vi "Fixed-Point Multirate Filter Modeling and Simulation.vi"() -> ()   [LabVIEW 2023]
doc: "Demonstrates how to use the DFD FXP MRate Modeling VI and the DFD FXP MRate Simulation VI to model and simulate the behavior of a fixed-point multirate filter, respectively."
uses:
  <vilib>/addons/Digital Filter Design/_Objects.llb/DFD Quantization Settings.ctl
  <vilib>/addons/Digital Filter Design/_Objects.llb/DFD Quantization Sources.ctl
  <vilib>/addons/Digital Filter Design/Design.llb/DFD MRate Filter Design (Integer).vi
  <vilib>/addons/Digital Filter Design/FXPMRateSim.llb/DFD FXP MRate Simulation (DBL).vi
  <vilib>/addons/Digital Filter Design/Multirate.llb/DFD MRate Filtering (Array).vi
  <vilib>/Analysis/NI_AALBase.lvlib
  <vilib>/addons/Digital Filter Design/NI_DigFilterLicensed.lvlib
  <vilib>/Analysis/NI_AALPro.lvlib
panel:
  out "MSE":dbl format="%.6g"
  out "Error Message":string
  out "Filtered Signals":dbl[][](graph)
  in  "Output Word Length":i16=16
  in  "Input Word Length":i16=16
  in  "Coefficients Word Length":i16=16
  in  "Source":enum16{"Sine", "Random Noise"}(ring)
  in  "Number of Samples":i32=128
  # "Select Help>>Show Context Help and move the cursor over the VI icon for more information."
  # "Quantization Setting"
  # "Signal Settings"
  # "Modeling Settings"
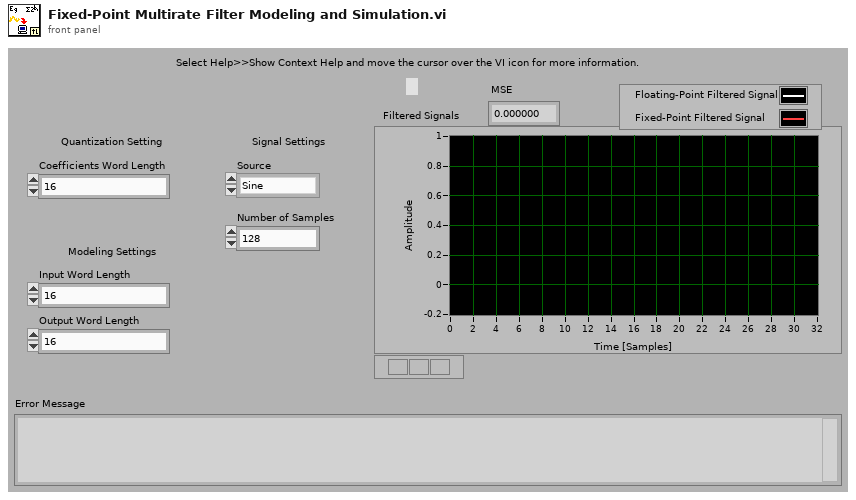
[diagram p1: front panel]
types:
  T1 = typedef "NI_DigFilterLicensed.lvlib/DFD Quantization Settings.ctl" = cluster{"source":T2, "wl":i16, "iwl":i16, "overflow mode":enum16{"Saturation", "Wrap"}, "rounding mode":enum16{"Nearest", "Truncation"}, "signed?":bool}
  T2 = typedef "NI_DigFilterLicensed.lvlib/DFD Quantization Sources.ctl" = u16
  T3 = typedef "NI_DigFilterLicensed.lvlib/DFD Multirate Filter Obj.ctl" = cluster{"mMRate_Structure":enum16{"CIC", "FIR", "IIR", "Lattice"}, "mMRate_Mode":T4, "mMRate_Factor":i32, "mMRate_FIRParams":cluster{"mMRate_FIR_H":dbl[], "mMRate_FIR_IsNyquist?":bool, "mMRate_FIR_IsSymmetric?":bool}, "mMRate_CICParams":cluster{"mMRate_CIC_#Stage":i32, "mMRate_CIC_Lag":i32, "mMRate_CIC_Type":enum16{"Lowpass", "Highpass"}}, "mMRate_Order":i32, "mMRate_Version":string, "mMRate_Comments":string, "mMRate_RationalFactor":cluster{"mMRate_L":i32, "mMRate_M":i32}, "mMRate_Fs":dbl, "mMRate_Quantized?":bool, "mMRate_QFilterGain":dbl, "mMRate_CoefWl":i16, "mMRate_Scaling":cluster{"mMRate_ScaleByPowerOf2?":bool, "mMRate_ScaleType":T5}, "mMRate_InputWl":i16, "mMRate_OutputWl":i16, "mMRate_OutputMode":T6, "mMRate_MultMode":T7, "mMRate_BitPruning":bool, "mMRate_GainWl":i16, "mMRate_OutputFwl":i16, "mMRate_SumIwl":i16, "mMRate_InputIwl ":i16, "mMRate_SumWl":i16, "mMRate_CoefIwl":i16}
  T4 = typedef "NI_DigFilterLicensed.lvlib/DFD Multirate Mode.ctl" = i16
  T5 = typedef "NI_DigFilterLicensed.lvlib/DFD Coef Norm Type.ctl" = enum16{"No Norm", "Time Domain 1-Norm", "Time Domain 2-Norm", "Time Domain Inf-Norm"}
  T6 = typedef "NI_DigFilterLicensed.lvlib/DFD Round-off Mode.ctl" = enum16{"Nearest", "Truncation"}
  T7 = typedef "NI_DigFilterLicensed.lvlib/DFD FXP MRate Multiply Mode.ctl" = enum16{"Truncated", "Full"}
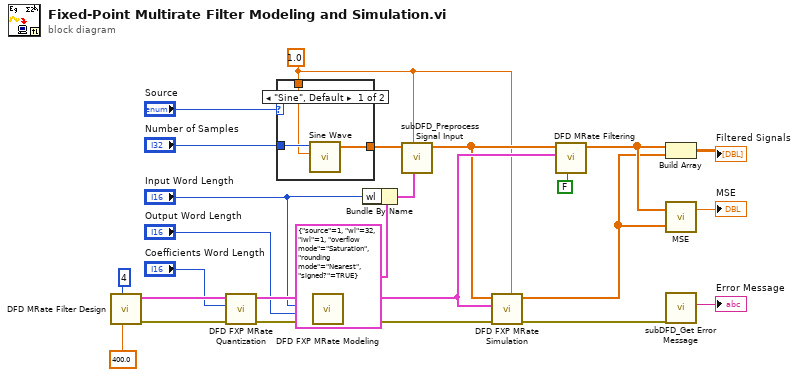
[diagram p0: block diagram]
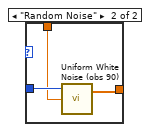
[diagram p2: hidden frame]
diagram:
  w1 = 1.0 ("input range")
  n1 = call-poly <vilib>:"DFD MRate Filter Design.vi"("fs in [Hz]"=400.0, "factor"=4) -> ("error out"=w24:errorcluster, "multirate filter out"=w25:T3)  [unwired: 6 in, 2 out]
  n2 = call <vilib>:"DFD FXP MRate Quantization.vi"("error in (no error)"=w24, "coefficients word length"="Coefficients Word Length", "multirate filter in"=w25) -> ("error out"=w20:errorcluster, "multirate filter out"=w21:T3)  [unwired: 3 in, 4 out]
  n3 = case shown="\"Sine\", Default" "Source" {
    tunnel: [w28 w30] -> w10
    tunnel: "Number of Samples" -> [w27 w31]
    tunnel: w1 -> [w26 w29]
    frame "Sine", Default {
      n4 = call <vilib>:"Sine Wave.vi"("samples"=w27, "amplitude"=w26) -> ("sine wave"=w28:dbl[])  [unwired: 3 in, 2 out]
    }
    frame "Random Noise" {
      n5 = call <vilib>:"Uniform White Noise (obs 90).vi"("amplitude"=w29, "samples"=w31) -> ("uniform white noise"=w30:dbl[])  [unwired: 1 in, 1 out]
    }
  }
  n6 = call <vilib>:"DFD FXP MRate Modeling.vi"("error in (no error)"=w20, "output word length"="Output Word Length", "input word length"="Input Word Length", "multirate filter in"=w21) -> ("error out"=w18:errorcluster, "multirate filter out"=w17:T3)  [unwired: 4 in, 2 out]
  n7 = Bundle By Name(cluster=T1 {"source"=1, "wl"=32, "iwl"=1, "overflow mode"=enum."Saturation", "rounding mode"=enum."Nearest", "signed?"=TRUE} ("input quantizer"), "wl"="Input Word Length") -> (w6:T1)
  n8 = call <vilib>:"subDFD_Preprocess Signal Input.vi"("input quantizer"=w6, "input range"=w1, "x"=w10) -> ("q[x]"=w9:dbl[])  [unwired: 8 out]
  n9 = call-poly <vilib>:"DFD FXP MRate Simulation.vi"("input range"=w1, "error in (no error)"=w18, "multirate filter"=w17, "signal in"=w9) -> ("error out"=w11:errorcluster, "DBL signal out"=w4:dbl[])  [unwired: 1 in, 5 out]
  n10 = call-poly <vilib>:"DFD MRate Filtering.vi"("zero phase? (T)"=FALSE, "multirate filter"=w17, "signal in"=w9) -> ("signal out"=w5:dbl[])  [unwired: 2 in, 6 out]
  n11 = Build Array(w5, w4) -> (→"Filtered Signals":dbl[][])
  n12 = call <vilib>:"MSE.vi"("X Values"=w4, "Y Values"=w5) -> ("mse"=→"MSE":dbl)  [unwired: 1 out]
  n13 = call <vilib>:"subDFD_Get Error Message.vi"("error in (no error)"=w11) -> ("Error Message"=→"Error Message":string)  [unwired: 10 out]
